vi "test.vi"() -> ()   [LabVIEW 2015]
panel:
  in  "Read data":string="RD"
  in  "Write data":string="WD"
  out "error out":errorcluster
  in  "Write":bool
  in  "COM":refnum<visa-resource-name>="COM5"
  in  "Beginning Words":u16 max=9999 format="%04.0f"
  in  "Number of Data":u16=1 format="%0.0f"
  out "Read Data":u32[](array[numeric])
  in  "Write Data":i32[](array[numeric])=[1, 2, 3, 4, 5, 6, 7, 8, 9, 0] max=9999 format="%04.0f"
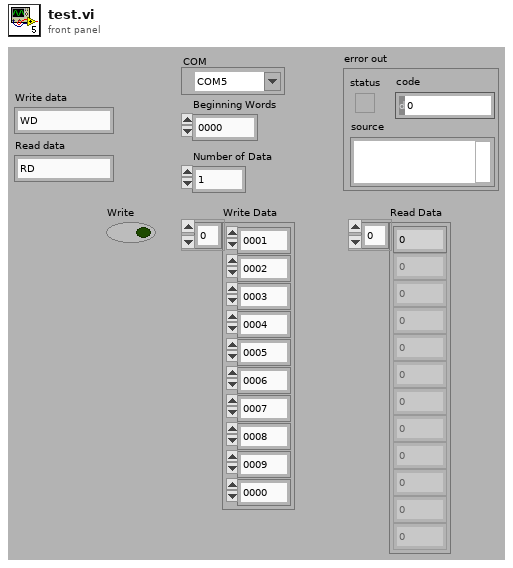
[diagram p1: front panel]
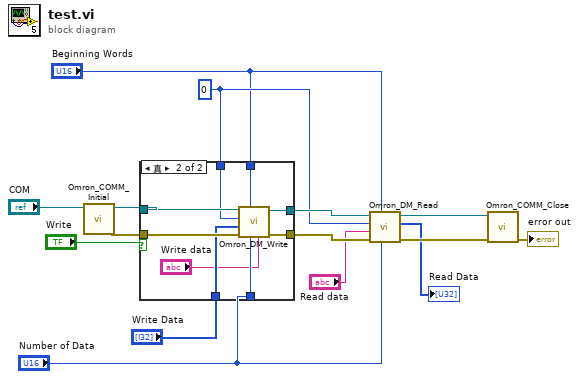
[diagram p0: block diagram]
diagram:
  w9 = u8 0 ("Unit No.")
  n1 = call "Omron_COMM_Initial.vi"("COM in"="COM") -> ("error out"=w13:errorcluster, "COM out"=w14:refnum<visa-resource-name>)  [unwired: 9 in]
  n2 = case shown="真" "Write" {
    tunnel: w14 -> [w17 w26]
    tunnel: w13 -> [w16 w25]
    tunnel: "Write Data" -> [_ w24]
    tunnel: [w17 w23] -> w11
    tunnel: [w16 w22] -> w10
    tunnel: w9 -> [_ w21]
    tunnel: "Beginning Words" -> [_ w20]
    tunnel: "Number of Data" -> [_ w19]
    frame False {
    }
    frame True {
      n3 = call "Omron_DM_Write.vi"("Command"="Write data", "Number of Data"=w19, "Beginning Words"=w20, "error in"=w25, "Write Data"=w24, "Unit No."=w21, "COM in"=w26) -> ("error out"=w22:errorcluster, "COM out"=w23:refnum<visa-resource-name>)  [unwired: 3 in]
    }
  }
  n4 = call "Omron_DM_Read.vi"("No of Words"="Number of Data", "Beginning Words"="Beginning Words", "error in"=w10, "Command"="Read data", "Unit No."=w9, "COM in"=w11) -> ("error out"=w5:errorcluster, "Read Data"=→"Read Data":u32[], "COM out"=w6:refnum<visa-resource-name>)  [unwired: 3 in]
  n5 = call "Omron_COMM_Close.vi"("error in"=w5, "COM in"=w6) -> ("error out"=→"error out":errorcluster)  [unwired: 9 in]
